vi "Rotation3d_Equals.vi"(9 "other Rotation3d":T1={"Q_quaternion"={"R"=1.0, "V"=[0.0, 0.0, 0.0]}}, 11 "in Rotation3d":T1={"Q_quaternion"={"R"=1.0, "V"=[0.0, 0.0, 0.0]}}) -> (3 "Equals":bool)   [LabVIEW 2019, in "Trajectory_Library.lvlib"]
doc: "Adds two rotations together, with the result being bounded between -pi and pi.\n\nFor example, Rotation2d.fromDegrees(30) + Rotation2d.fromDegrees(60) = Rotation2d{-pi/2}\n\nThis function is the same as RotateBy.\n\nParameters:\n\n - IN ROTATION - This rotation data structure\n - OTHER ROTATION - The rotation to add.\n\nReturns:\n- OUT ROTATION - The sum of the two rotations."
uses:
  Trajectory_Library.lvlib
  ROTATION3D.ctl
  QUATERNION.ctl
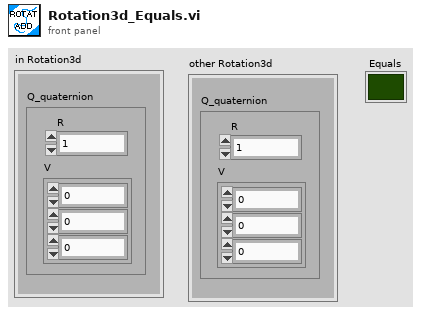
[diagram p1: front panel]
types:
  T1 = typedef "Trajectory_Library.lvlib/ROTATION3D.ctl" = cluster{"Q_quaternion":T2}
  T2 = typedef "Trajectory_Library.lvlib/QUATERNION.ctl" = cluster{"R":dbl, "V":dbl[]}
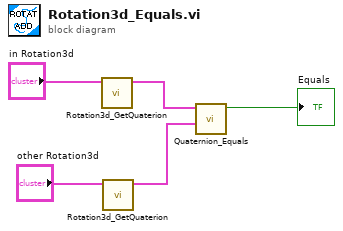
[diagram p0: block diagram]
diagram:
  n1 = call "Rotation3d_GetQuaterion.vi"("in Rotation3d"="in Rotation3d") -> ("out Quaterion"=w3:T2)  [unwired: 10 in]
  n2 = call "Rotation3d_GetQuaterion.vi"("in Rotation3d"="other Rotation3d") -> ("out Quaterion"=w2:T2)  [unwired: 10 in]
  n3 = call "Quaternion_Equals.vi"("Other Quaternion"=w2, "Quaternion"=w3) -> ("Equal"=→"Equals":bool)  [unwired: 8 in, 1 out]
